vi "LF_Tester_RCstage_dbTester_v2.vi"(0 "string":string, 1 "Current(A) Input":dbl=291.8 format="%#_13g", 3 "Emitter Image Data":path=path "O:/PT_Projects/DT18/57_Testing/X57-0LT_LifeTester_Proj/LabVIEW_prog/TestData/20190514_RClinearStageTest/emitter.txt", 4 "Power Meter Data File":path=path "O:/PT_Projects/DT18/57_Testing/X57-0LT_LifeTester_Proj/LabVIEW_prog/TestData/20190514_RClinearStageTest/power.txt", 5 "Number of Spectrometers":i32, 6 "Wrapper In":u32, 7 "Power Meter":enum16{"Front", "Back"}(ring), 9 "Spectrometer":enum16{"Front", "Back"}(ring), 10 "Spectrometer Data File":path=path "O:/PT_Projects/DT18/57_Testing/X57-0LT_LifeTester_Proj/LabVIEW_prog/TestData/20190514_RClinearStageTest/spectrum.txt", 11 "Illasco_SN":string[](array[string])=["LF_15", "LF_14", "LF_13", "LF_12", "LF_11", "LF_10", "LF_9", "LF_8", "LF_7", "LF_6", "LF_5", "LF_4", "LF_3", "LF_2", "LF_1"], 12 "Select Camera":T1="lfCam_Front", 14 "Stage Ref. In":refnum<visa-resource-name>="Lf_Tester_Stage_Front", 15 "Stop data acquisition":bool) -> ()   [LabVIEW 2017]
doc: "Use this template to build a simple state machine design pattern. Each state executes code and determines which state to transition to."
uses:
  <vilib>/userdefined/High Color/IMAQdx.ctl
  State.ctl
  <vilib>/vision/driver/NI_Vision_Acquisition_Software.lvlib
panel:
  out "Emitter Count":i32=15
  out "Start time":timestamp=timestamp(3640692023.4345794 s since 1904-01-01)
  out "Power(W)":dbl=-0.1 format="%.2f"
  out "Dataset #":i32=34
  in  "Automatic Life Tester by Chao Gong":enum32{"Spectrometer", "Pixelink Cam"}(tab)
  out "Background":dbl=-2.39316239316236
  in  "Ocean Spectrometer Input":T2={"Boxcar"=1.0, "Average"=1.0, "Integration (ms)"=100.0} {"Integration (ms)" min=1.0 max=1000.0 step=1.0 format="%#_2f"; "Average" min=1.0 max=1000.0 step=1.0; "Boxcar" min=1.0 max=1000.0 step=1.0}
  out "Centroid_Wavelength(nm)":dbl=907.813706851305
  out "Ocean Optics Spectrometer":T3(graph)
  out "Bar Emitter Image":T4(plugin-control)
  # "Initialization"
  # "Instructions:\n1. Choose stage from stage ref. in\n2. Choose power meter\n3. Choose spectrometer \n4. Select camera\n5. Choose folder directory to save data\n6. Name illasco SN number. Num 1 on the most right side\n7. Change current input value based on running condition."
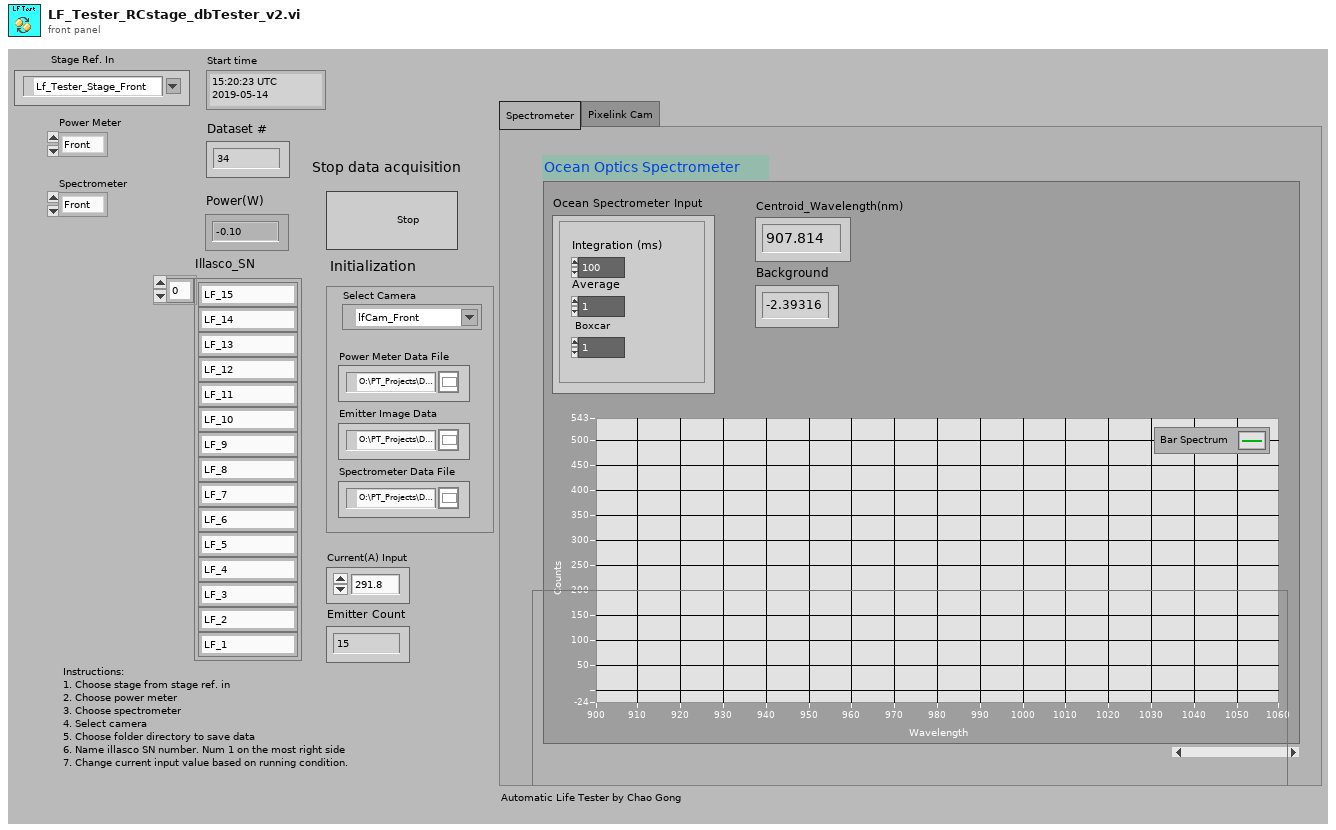
[diagram p1: front panel]
types:
  T1 = typedef "IMAQdx.ctl" = refnum<k21>
  T2 = cluster{"Boxcar":dbl, "Average":dbl, "Integration (ms)":dbl}
  T3 = cluster{"WL Values":dbl[], "Spectrum Values":dbl[]}
  T4 = typedef "IMAQ Image.ctl" = refnum<image>
  T5 = typedef "State.ctl" = enum16{"Take and Save Power Data", "Take and Save Emitter Image", "Take and Save Spectrometer Data", "Move Translational Stage"}
  T6 = typedef "Image Type" = u32
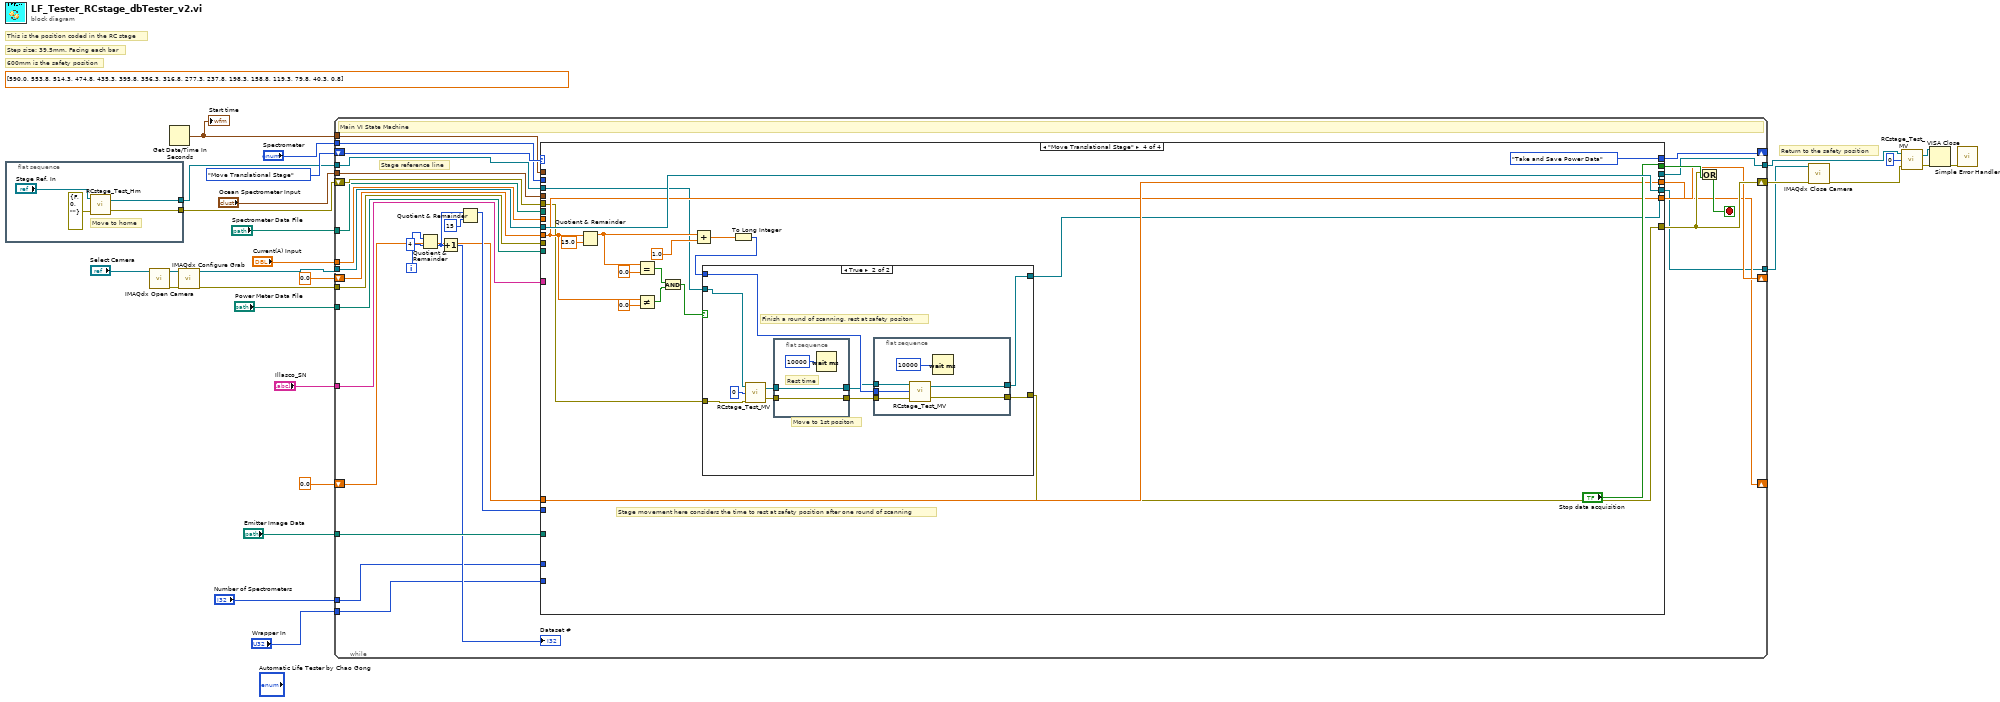
[diagram p0: block diagram]
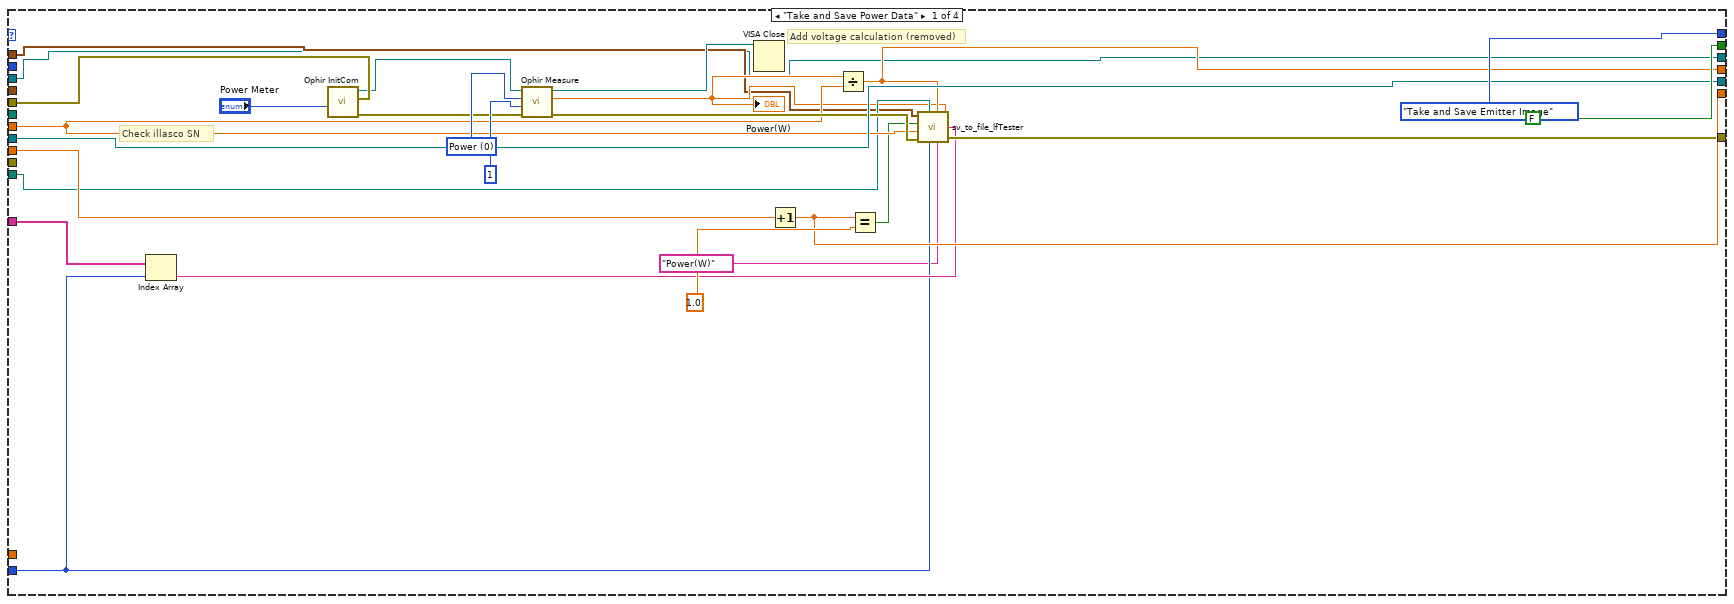
[diagram p2: hidden frame]
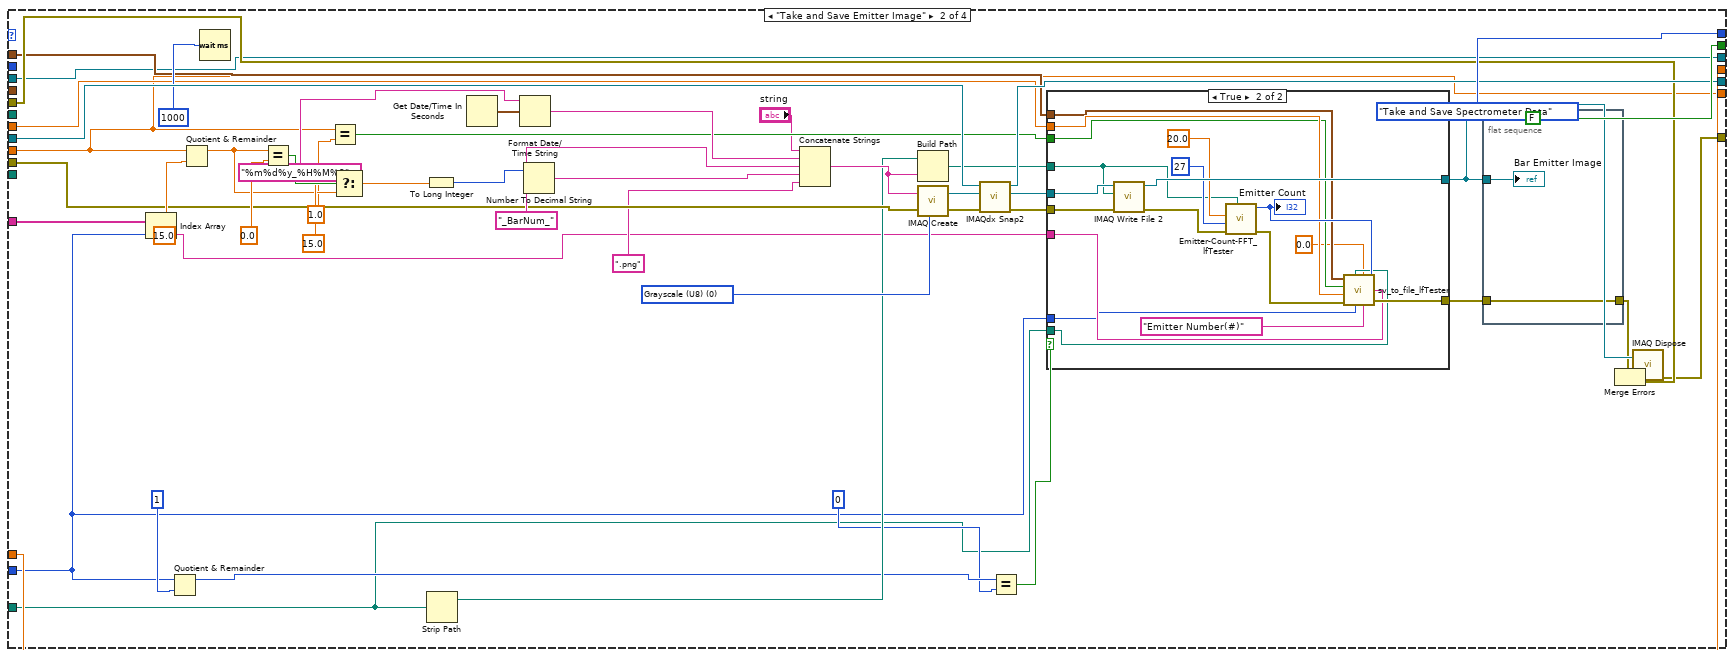
[diagram p3: hidden frame]
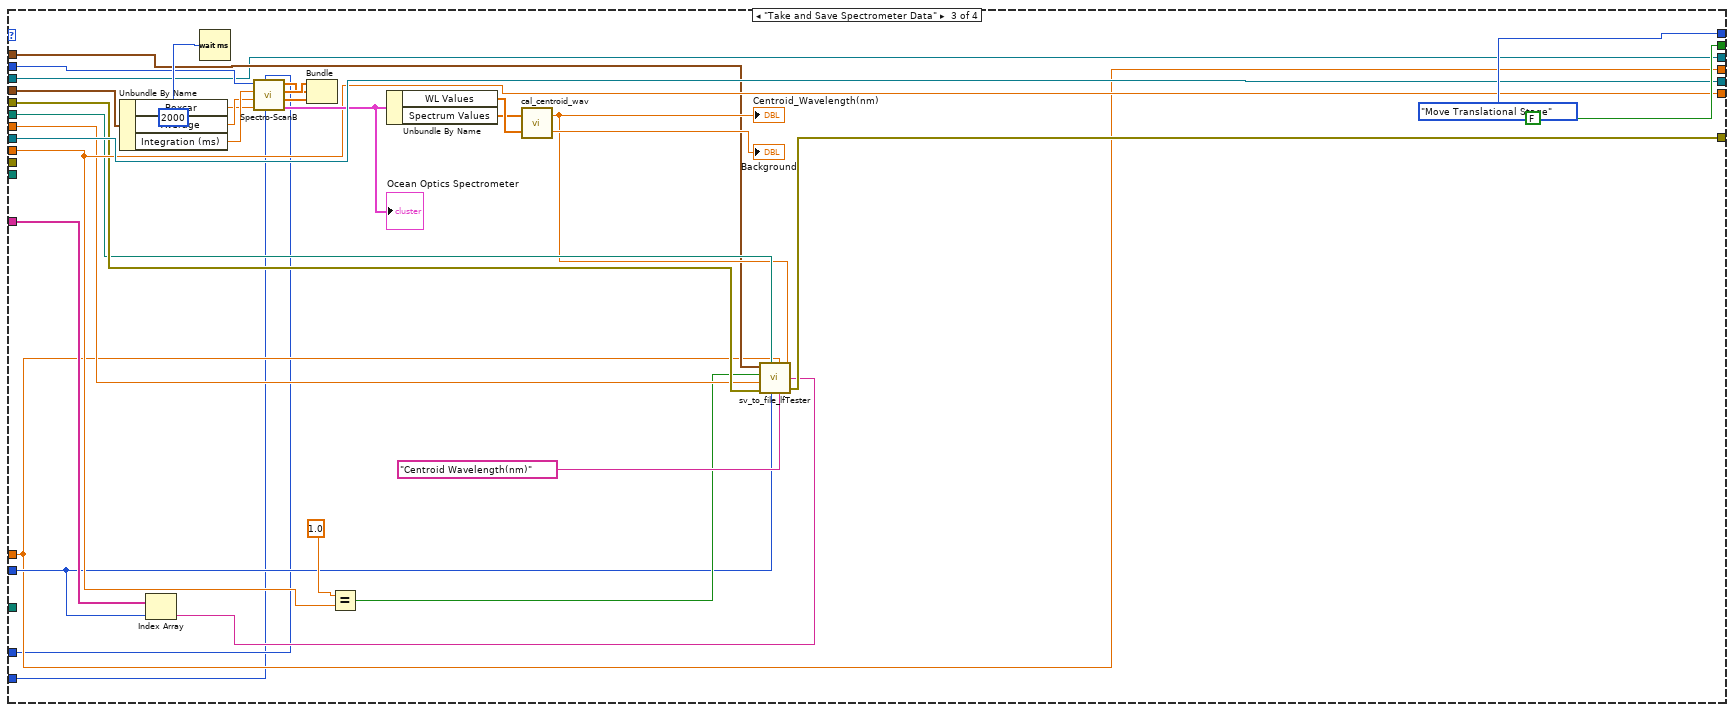
[diagram p5: hidden frame]
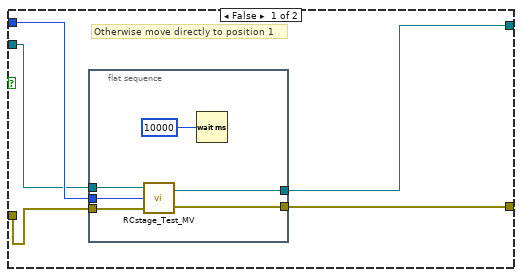
[diagram p6: hidden frame]
diagram:
  (unwired) dbl[] [590.0, 553.8, 514.3, 474.8, 435.3, 395.8, 356.3, 316.8, 277.3, 237.8, 198.3, 158.8, 119.3, 79.8, 40.3, 0.8] ("Linear Stage Moving Position")
  # "This is the position coded in the RC stage"
  # "600mm is the safety position"
  # "Step size: 39.5mm. Facing each bar"
  # "Return to the safety position"
  n1 = flat-sequence {
    tunnel: [w29] -> w12
    tunnel: [w30] -> w10
    frame #0 {
      # "Move to home"
      n2 = call "RCstage_Test_Hm.vi"("error in"=errorcluster {"status"=FALSE, "code"=0, "source"=""}, "Stage Ref.  In"="Stage Ref. In") -> ("error out"=w29:errorcluster, "Stage Ref. Out"=w30:refnum<visa-resource-name>)  [unwired: 1 in]
    }
  }
  n3 = call <vilib>:"IMAQdx Open Camera.vi"("Session In"="Select Camera") -> ("error out"=w24:errorcluster, "Session Out"=w25:T1)  [unwired: 9 in]
  n4 = Get Date/Time In Seconds() -> (seconds since 1Jan1904=w16:timestamp)
  "Start time" <- w16
  n5 = call <vilib>:"IMAQdx Configure Grab.vi"("error in"=w24, "Session In"=w25) -> ("error out"=w23:errorcluster, "Session Out"=w19:T1)  [unwired: 8 in]
  n6 = while {
    shift-right: [w62] -> _
    shift-left: State."Move Translational Stage" ("Initial State") -> [w63]
    shift-right: [w59] -> w14
    shift-left: w12 -> [w61]
    shift-right: [w56] -> _
    shift-left: 0.0 ("x") -> [w57]
    tunnel: "Emitter Image Data" -> [w54]
    tunnel: w23 -> [w53]
    tunnel: "Ocean Spectrometer Input" -> [w52]
    tunnel: "Spectrometer Data File" -> [w51]
    tunnel: "Current(A) Input" -> [w48]
    tunnel: "Illasco_SN" -> [w47]
    tunnel: w16 -> [w46]
    tunnel: "Power Meter Data File" -> [w45]
    shift-right: [w40] -> _
    shift-left: 0.0 -> [w37]
    tunnel: "Spectrometer" -> [w39]
    tunnel: "Number of Spectrometers" -> [w34]
    tunnel: w10 -> [w38]
    tunnel: [w35] -> w3
    tunnel: w19 -> [w55]
    tunnel: [w36] -> w4
    tunnel: "Wrapper In" -> [w33]
    i -> [w50]
    stop <- w58 stop-if-true
    # "Stage reference line"
    # "Main VI State Machine"
    n7 = Quotient & Remainder(x=w50, y=4) -> (floor(x/y)=w42:i32)  [unwired: 1 out]
    n8 = Increment(x=w42) -> (x+1=→"Dataset #":i32)
    n9 = Quotient & Remainder(x=w42, y=15) -> (x-y*floor(x/y)=w41:i32)  [unwired: 1 out]
    n10 = case shown="\"Move Translational Stage\"" w63 {
      tunnel: [State."Take and Save Emitter Image" ("Next State") State."Take and Save Spectrometer Data" ("Next State") State."Move Translational Stage" ("(Value Not Used)") State."Take and Save Power Data" ("Initial State")] -> w62
      tunnel: [FALSE ("Stop Loop?") FALSE ("Stop Loop?") FALSE ("Stop Loop?") "Stop data acquisition"] -> w60
      tunnel: w61 -> [w84 w120 w173 w197]
      tunnel: [w76 w119 w175 w194] -> w59
      tunnel: w57 -> [w81 w92 w177 w203]
      tunnel: [w77 w92 w177 w203] -> w56
      tunnel: w55 -> [w79 w136 w191 w211]
      tunnel: w54 -> [_ w96 _ _]
      tunnel: w53 -> [_ w125 _ _]
      tunnel: [w79 w123 w191 w211] -> w36
      tunnel: w52 -> [_ _ w189 _]
      tunnel: w51 -> [_ _ w171 _]
      tunnel: w48 -> [w72 w100 w169 _]
      tunnel: w47 -> [w78 w95 w178 _]
      tunnel: w46 -> [w68 w97 w168 _]
      tunnel: w45 -> [w70 _ _ _]
      tunnel: w41 -> [w73 w93 w166 _]
      tunnel: [w71 w102 w164 w208] -> w40
      tunnel: w37 -> [_ w102 w164 w208]
      tunnel: w39 -> [_ _ w165 _]
      tunnel: w38 -> [w64 w91 w163 w198]
      tunnel: [w64 w91 w163 w195] -> w35
      tunnel: w34 -> [_ _ w162 _]
      tunnel: w33 -> [_ _ w161 _]
      frame "Take and Save Power Data" {
        w87 = u16 0 items=["Power", "Energy", "Frequency"] ("Measure Choice (0:Power)")
        # "Add voltage calculation (removed)"
        # "Check illasco SN"
        # "User State 1 - Replace this state with functionality for your own application."
        n11 = Index Array(array=w78, index=w73) -> (element=w74:string)
        n12 = call "Ophir InitCom.vi"("error in (no error)"=w84, "USB Channel number (default 0)"="Power Meter") -> ("error out"=w83:errorcluster, "dup Visa Session"=w82:refnum<visa-resource-name>)  [unwired: 5 in, 1 out]
        n13 = call "Ophir Measure.vi"("error in (no error)"=w83, "Power Method ?(0)"=1, "Measure Choice (0:Power)"=w87, "Visa Session"=w82) -> ("error out"=w75:errorcluster, "Value Number"=w69:dbl, "dup Visa Session"=w85:refnum<visa-resource-name>)  [unwired: 1 out]
        "Power(W)" <- w69
        n14 = VISA Close(VISA resource name=w85) -> ()  [unwired: 1 in, 1 out]
        n15 = Increment(x=w81) -> (x+1=w77:dbl)
        n16 = Divide(x=w69, y=w72) -> (x/y=w71:dbl)
        n17 = Equal?(x=w77, y=1.0) -> (x = y?=w67:bool)
        n18 = call "sv_to_file_lfTester.vi"("Test case"="Power(W)", "Illasco SN"=w74, "Measured Value"=w69, "Calculated voltage"=w71, "Dataset divide 15"=w73, "Error in"=w75, "Current(A) Input"=w72, "Data file directory"=w70, "Whether first line"=w67, "Start time"=w68) -> ("Error out"=w76:errorcluster)
      }
      frame "Take and Save Emitter Image" {
        w122 = T6 0 items=["Grayscale (U8)", "Grayscale (I16)", "Grayscale (SGL)", "Complex (CSG)", "RGB (U32)", "HSL (U32)", "RGB (U64)", "Grayscale (U16)"] ("Image Type")
        # "User State 2 - Replace this state with functionality for your own application."
        n19 = Index Array(array=w95, index=w93) -> (element=w94:string)
        n20 = Quotient & Remainder(x=w93, y=1) -> (x-y*floor(x/y)=w106:i32)  [unwired: 1 out]
        n21 = Quotient & Remainder(x=w92, y=15.0) -> (x-y*floor(x/y)=w129:dbl)  [unwired: 1 out]
        n22 = Wait (ms)(milliseconds to wait=u32 1000) -> ()  [unwired: 1 out]
        n23 = Equal?(x=w129, y=0.0) -> (x = y?=w131:bool)
        n24 = Equal?(x=w92, y=1.0) -> (x = y?=w98:bool)
        n25 = Select(t=15.0, s=w131, f=w129) -> (s? t:f=w128:dbl)
        n26 = To Long Integer(number=w128) -> (32bit integer=w127:i32)
        n27 = Strip Path(path=w96) -> (stripped path=w111:path)  [unwired: 1 out]
        n28 = Get Date/Time In Seconds() -> (seconds since 1Jan1904=w113:timestamp)
        n29 = Format Date/Time String(time format string (%c)="%m%d%y_%H%M%S", seconds (now)=w113) -> (date/time string=w108:string)  [unwired: 1 in]
        n30 = Number To Decimal String(number=w127) -> (decimal integer string=w134:string)  [unwired: 1 in]
        n31 = Concatenate Strings("string", w108, "_BarNum_" ("element"), w134, ".png" ("string")) -> (w114:string)
        n32 = Build Path(base path=w111, name or relative path=w114) -> (appended path=w116:path)
        n33 = call "IMAQ Create"("Image Name"=w114, "Image Type"=w122, "error in (no error)"=w125) -> ("New Image"=w126:T4, "error out"=w124:errorcluster)  [unwired: 2 in]
        n34 = call <vilib>:"IMAQdx Snap2.vi"("error in"=w124, "Image In"=w126, "Session In"=w136) -> ("error out"=w110:errorcluster, "Image Out"=w117:T4, "Session Out"=w123:T1)  [unwired: 6 in]
        n35 = Equal?(x=w106, y=0) -> (x = y?=w104:bool)
        n36 = case shown="True" w104 {
          tunnel: [w142 w160] -> w118
          tunnel: [w141 w151] -> w101
          tunnel: w117 -> [w142 w159]
          tunnel: w116 -> [_ w156]
          tunnel: w110 -> [w141 w155]
          tunnel: w100 -> [_ w149]
          tunnel: w98 -> [_ w148]
          tunnel: w97 -> [_ w147]
          tunnel: w96 -> [_ w146]
          tunnel: w94 -> [_ w144]
          tunnel: w93 -> [_ w143]
          frame False {
          }
          frame True {
            n37 = call-poly "IMAQ Write File 2"("error in (no error)"=w155, "File Path"=w156, "Image"=w159) -> ("error out"=w154:errorcluster, "Image Out (duplicate)"=w160:T4)  [unwired: 7 in]
            n38 = call "Emitter-Count-FFT_lfTester.vi"("Bar Image Path"=w156, "Error In"=w154, "Emitter #"=27, "Threshold (%)"=20.0) -> ("Error Out"=w152:errorcluster, "Emitter Count"=w150:i32)  [unwired: 1 in, 2 out]
            "Emitter Count" <- w150
            n39 = call "sv_to_file_lfTester.vi"("Test case"="Emitter Number(#)", "Illasco SN"=w144, "Measured Value"=w150, "Calculated voltage"=0.0, "Dataset divide 15"=w143, "Error in"=w152, "Current(A) Input"=w149, "Data file directory"=w146, "Whether first line"=w148, "Start time"=w147) -> ("Error out"=w151:errorcluster)
          }
        }
        n40 = flat-sequence {
          tunnel: w118 -> [w140]
          tunnel: w101 -> [w139]
          tunnel: [w139] -> w103
          frame #0 {
            "Bar Emitter Image" <- w140
          }
        }
        n41 = call "IMAQ Dispose"("Image"=w118, "error in (no error)"=w103) -> ("error out"=w121:errorcluster)  [unwired: 4 in]
        n42 = Merge Errors(w121, w120) -> (w119:errorcluster)
      }
      frame "Take and Save Spectrometer Data" {
        n43 = Unbundle By Name(w189) -> ("Boxcar"=w186:dbl, "Average"=w187:dbl, "Integration (ms)"=w188:dbl)
        n44 = Index Array(array=w178, index=w166) -> (element=w172:string)
        n45 = Wait (ms)(milliseconds to wait=u32 2000) -> ()  [unwired: 1 out]
        n46 = call "Spectro-ScanB.vi"("Wrapp in"=w161, "Spectrometer num"=w162, "Boxcar"=w186, "Average"=w187, "Integration (ms)"=w188, "Spectrometer Selection"=w165) -> ("Ocean Optics Spectrometer Single Scan Program"=w190:T3, "Spectral PowerBD"=w183:dbl[], "Spectral Power"=w185:dbl[], "Wavelength (nm)"=w184:dbl[])
        "Ocean Optics Spectrometer" <- w190
        n47 = Bundle("Spectral Power"=w185, "Wavelength (nm)"=w184, "Spectral PowerBD"=w183) -> ()  [unwired: 1 in, 1 out]
        n48 = Equal?(x=1.0, y=w177) -> (x = y?=w167:bool)
        n49 = Unbundle By Name(w190) -> ("WL Values"=w180:dbl[], "Spectrum Values"=w179:dbl[])
        n50 = call "cal_centroid_wav.vi"("Raw Wavelength data"=w180, "Raw Intensity Data"=w179) -> ("Background"=→"Background":dbl, "Centroid Wavelength"=w170:dbl)
        "Centroid_Wavelength(nm)" <- w170
        n51 = call "sv_to_file_lfTester.vi"("Test case"="Centroid Wavelength(nm)", "Illasco SN"=w172, "Measured Value"=w170, "Calculated voltage"=w164, "Dataset divide 15"=w166, "Error in"=w173, "Current(A) Input"=w169, "Data file directory"=w171, "Whether first line"=w167, "Start time"=w168) -> ("Error out"=w175:errorcluster)
      }
      frame "Move Translational Stage" {
        # "Stage movement here considers the time to rest at safety position after one round of scanning"
        n52 = Quotient & Remainder(x=w203, y=15.0) -> (x-y*floor(x/y)=w205:dbl)  [unwired: 1 out]
        n53 = Equal?(x=w205, y=0.0) -> (x = y?=w201:bool)
        n54 = Not Equal?(x=w203, y=0.0) -> (x != y?=w200:bool)
        n55 = And(x=w201, y=w200) -> (x .and. y?=w199:bool)
        n56 = Add(x=w205, y=1.0) -> (x+y=w206:dbl)
        n57 = To Long Integer(number=w206) -> (32bit integer=w196:i32)
        n58 = case shown="True" w199 {
          tunnel: w198 -> [w216 w233]
          tunnel: w197 -> [w215 w231]
          tunnel: w196 -> [w217 w228]
          tunnel: [w213 w225] -> w195
          tunnel: [w214 w224] -> w194
          frame False {
            # "Otherwise move directly to position 1"
            n59 = flat-sequence {
              tunnel: w217 -> [w222]
              tunnel: w216 -> [w221]
              tunnel: w215 -> [w220]
              tunnel: [w219] -> w214
              tunnel: [w218] -> w213
              frame #0 {
                n60 = call "RCstage_Test_MV.vi"("error in"=w220, "Pos. Index"=w222, "Stage Ref. In"=w221) -> ("error out"=w219:errorcluster, "Stage Ref. Out"=w218:refnum<visa-resource-name>)
                n61 = Wait (ms)(milliseconds to wait=u32 10000) -> ()  [unwired: 1 out]
              }
            }
          }
          frame True {
            # "Move to 1st positon"
            # "Finish a round of scanning, rest at safety positon"
            n62 = call "RCstage_Test_MV.vi"("error in"=w231, "Pos. Index"=0, "Stage Ref. In"=w233) -> ("error out"=w230:errorcluster, "Stage Ref. Out"=w229:refnum<visa-resource-name>)
            n63 = flat-sequence {
              tunnel: w230 -> [w240]
              tunnel: w229 -> [w242]
              tunnel: [w242] -> w227
              tunnel: [w240] -> w226
              frame #0 {
                # "Rest time"
                n64 = Wait (ms)(milliseconds to wait=u32 10000) -> ()  [unwired: 1 out]
              }
            }
            n65 = flat-sequence {
              tunnel: w228 -> [w239]
              tunnel: w227 -> [w238]
              tunnel: w226 -> [w237]
              tunnel: [w236] -> w225
              tunnel: [w235] -> w224
              frame #0 {
                n66 = call "RCstage_Test_MV.vi"("error in"=w237, "Pos. Index"=w239, "Stage Ref. In"=w238) -> ("error out"=w235:errorcluster, "Stage Ref. Out"=w236:refnum<visa-resource-name>)
                n67 = Wait (ms)(milliseconds to wait=u32 10000) -> ()  [unwired: 1 out]
              }
            }
          }
        }
      }
    }
    n68 = Or(x=w59, y=w60) -> (x .or. y?=w58:bool)
  }
  n69 = call <vilib>:"IMAQdx Close Camera.vi"("error in"=w14, "Session In"=w4) -> ("error out"=w9:errorcluster)  [unwired: 9 in]
  n70 = call "RCstage_Test_MV.vi"("error in"=w9, "Pos. Index"=0, "Stage Ref. In"=w3) -> ("error out"=w6:errorcluster, "Stage Ref. Out"=w7:refnum<visa-resource-name>)
  n71 = VISA Close(VISA resource name=w7, error in (no error)=w6) -> (error out=w11:errorcluster)
  n72 = call <vilib>:"Simple Error Handler.vi"("error in (no error)"=w11) -> ()  [unwired: 4 in, 5 out]
